vi "Get Candidate Test Info.vi"(0 "Candidate ID":string, 11 "error in (no error)":errorcluster) -> (4 "Cluster":T1, 15 "error out":errorcluster)   [LabVIEW 2014, in "Coding Platform.lvlib"]
uses:
  Coding Platform.lvlib
  Datatypes/Candidate Test Info.ctl
  Typedefs/User Event Operations.ctl
  Datatypes/Candidate Test Info Query.ctl
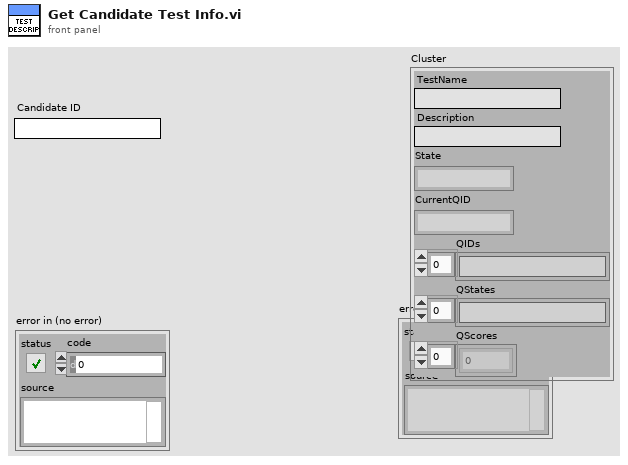
[diagram p1: front panel]
types:
  T1 = typedef "Coding Platform.lvlib/Candidate Test Info.ctl" = cluster{"TestName":string, "Description":string, "State":string, "CurrentQID":string, "QIDs":string[], "QStates":string[], "QScores":u64[]}
  T2 = typedef "Coding Platform.lvlib/Candidate Test Info Query.ctl" = cluster{"Candidate_ID":string, "notifier":refnum<notifier>}
  T3 = typedef "Coding Platform.lvlib/User Event Operations.ctl" = enum16{"Create", "Genereate", "Destroy", "Get Reference"}
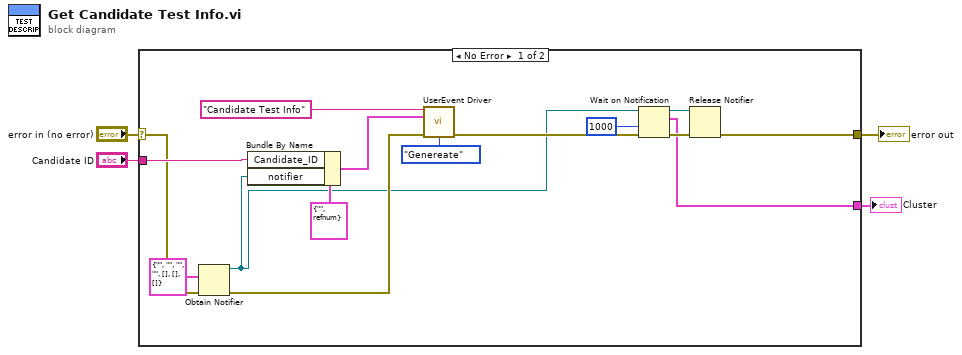
[diagram p0: block diagram]
diagram:
  n1 = case shown="No Error" "error in (no error)" {
    selector: "error in (no error)" -> [w7 w20]
    tunnel: [w11 w20] -> w4
    tunnel: "Candidate ID" -> [w14 _]
    tunnel: [w9 _] -> w1
    frame No Error {
      n2 = Obtain Notifier(notification data type=T1 {"TestName"="", "Description"="", "State"="", "CurrentQID"="", "QIDs"=[], "QStates"=[], "QScores"=[]}, error in (no error)=w7) -> (notifier out=w5:refnum<notifier>, error out=w8:errorcluster)  [unwired: 2 in, 1 out]
      n3 = Bundle By Name(cluster=T2 {"Candidate_ID"="", "notifier"=refnum} ("Login"), "Candidate_ID"=w14, "notifier"=w5) -> (w15:T2)
      n4 = call "UserEvent Driver.vi"("Message"="Candidate Test Info", "Data"=w15, "error in (no error)"=w8, "Operations(Get Reference)"=User_Event_Operations."Genereate") -> ("error out"=w19:errorcluster)  [unwired: 10 in, 1 out]
      n5 = Wait on Notification(notifier=w5, timeout in ms (-1)=1000, error in (no error)=w19) -> (notifier out=w10:refnum<notifier>, notification=w9:T1, error out=w13:errorcluster)  [unwired: 1 in, 1 out]
      n6 = Release Notifier(notifier=w10, error in (no error)=w13) -> (error out=w11:errorcluster)  [unwired: 1 in, 2 out]
    }
    frame Error {
    }
  }
  "error out" <- w4
  "Cluster" <- w1
